vi "LCD Retarder.vi"(8 "error in":errorcluster, 10 "Init Retardance (832nm)":dbl[unit]=8.32e-07, 11 "LCD In":refnum<class "LCD Retarder.lvclass">) -> (0 "errorOUT":errorcluster, 3 "LCD out":refnum<class "LCD Retarder.lvclass">)   [LabVIEW 2009, in "LCD Retarder.lvclass"]
uses:
  LCD Retarder.lvclass
  LCD Retarder.lvclass/LCD Retarder.ctl
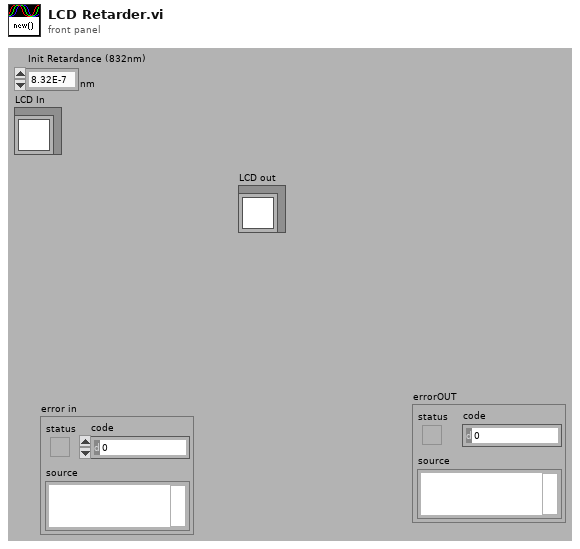
[diagram p1: front panel]
types:
  T1 = cluster{"Device Handle":u32, "Pipe 0 Handle":u32, "Pipe 1 Handle":u32}[]
  T2 = cluster{"Device Handle":u32, "Pipe 0 Handle":u32, "Pipe 1 Handle":u32}
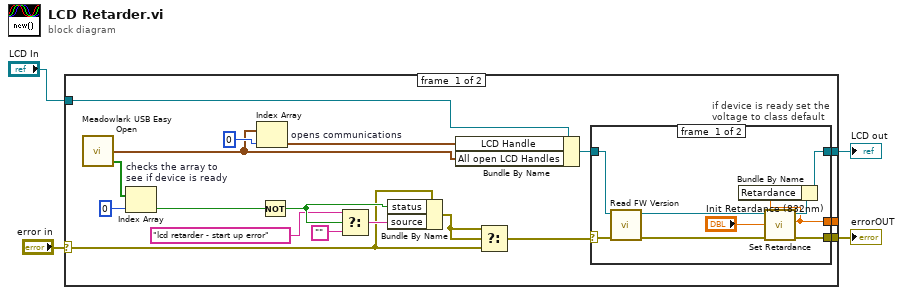
[diagram p0: block diagram]
diagram:
  n1 = case shown="No Error" "error in" {
    selector: "error in" -> [w5 w34]
    tunnel: [w22 w35] -> w4
    tunnel: "LCD In" -> [w21 w35]
    tunnel: [w20 _] -> _
    tunnel: [w18 w34] -> w2
    frame #0 {
      n2 = call "Meadowlark USB Easy Open.vi"() -> ("Device Opened Array"=w13:bool[], "USB Device and Pipes Array"=w8:T1)  [unwired: 1 out]
      n3 = Index Array "checks the array to\nsee if device is ready"(array=w13, index=0) -> (element=w19:bool)
      n4 = Index Array "opens communications"(array=w8, index=0) -> (element=w9:T2)
      n5 = Not(x=w19) -> (.not. x?=w16:bool)
      n6 = Select(t="lcd retarder - start up error", s=w16, f="") -> (s? t:f=w17:string)
      n7 = Bundle By Name(cluster=w5, "status"=w16, "source"=w17) -> (w7:errorcluster)
      n8 = Bundle By Name(cluster=w21, "LCD Handle"=w9, "All open LCD Handles"=w8) -> (w10:refnum<class "LCD Retarder.lvclass">)
      n9 = Select(t=w7, s=w7, f=w5) -> (s? t:f=w6:errorcluster)
      n10 = case "if device is ready set the \nvoltage to class default" shown="No Error" w6 {
        selector: w6 -> [w28 w33]
        tunnel: [w31 w33] -> w18
        tunnel: [w24 _] -> w20
        tunnel: w10 -> [w30 w32]
        tunnel: [w25 w32] -> w22
        frame #0 {
          n11 = call "Read FW Version.vi"("errorIN"=w28, "LCD in"=w30) -> ("error out"=w27:errorcluster, "LCD out"=w26:refnum<class "LCD Retarder.lvclass">)  [unwired: 8 out]
          n12 = call "Set Retardance.vi"("errorIN"=w27, "Retardance"="Init Retardance (832nm)", "LCD in"=w26) -> ("errorOUT"=w31:errorcluster, "Retardance out"=w24:dbl[unit], "LCD out"=w29:refnum<class "LCD Retarder.lvclass">)  [unwired: 6 out]
          n13 = Bundle By Name(cluster=w29, "Retardance"=w24) -> (w25:refnum<class "LCD Retarder.lvclass">)
        }
        frame #1 {
        }
      }
    }
    frame #1 {
    }
  }
  "LCD out" <- w4
  "errorOUT" <- w2
